vi "_LoPower_opt_fx.vi"(8 "ｘ":dbl, 9 "_LO_P_OPT":T1={"範囲配列"=[{"Start"=1.0, "Stop"=4.0, "Step"=0.05, "ｂｙ"="NEL VG"}, {"Start"=0.0, "Stop"=100.0, "Step"=4.0, "ｂｙ"="Motor"}, {"Start"=0.0, "Stop"=2.5, "Step"=0.1, "ｂｙ"="WCA VD"}], "Optimize"=0, "file_name"="LP_914.0_Tmin_100519.csv", "Save?"=FALSE, "measure"=1, "current(uA)"=60.0, "wait(ms)"=0, "IFfrq(GHz)"=8.0, "aveg"=10, "SISparam option"=2} {"SISparam option" items=["Volt and Current", "Volt only"]; "measure" items=["Pmax (only HOT)", "Tmin (HOT/COLD)", "C current"]; "Optimize" items=["Sweep", "黄金分割"]; "範囲配列"."Step" format="%.2f"; "範囲配列"."Stop" format="%.2f"; "範囲配列"."Start" format="%.2f"}, 10 "Control":T2={"GPIB_ATT"="28", "6501Dev#"=1, "GPIB_SP"="18", "GPIB_PM"="13", "GPIB_DSA"="11", "GPIB_DMM (TPD)"="23", "GPIB_MPI"="2", "mortor設定"=[{"Axis"=0, "ID"=0, "HIspeed"=200.0, "LOspeed"=100.0, "ACCEL(ms)"=100.0, "Sratio"=50.0, "フリーラン\n"=TRUE, "文字列"="DSB HOT/COLD"}, {"Axis"=1, "ID"=0, "HIspeed"=4.0, "LOspeed"=4.0, "ACCEL(ms)"=100.0, "Sratio"=50.0, "フリーラン\n"=TRUE, "文字列"="SubMM Att"}], "DATAパス"=path "Z:/band10/Labview_ALMA/MIX95/test", "DBパス "=path "Z:/band10/Labview_ALMA/MIX95/test", "comment"="P1_Tmin", "ColdCarts"="003601", "Th"=295.0, "Tc"=77.0, "Set_SIS_volt"=2.1, "Offset"=0.0, "control"=0, "FreqLO"=800.0, "Set_Mag_Cur"=800.0, "MPI offset(mm)"=22.99, "HOT/COLD"=0} {"HOT/COLD" items=["DSB", "SBR", "GainComp"]; "control" items=["CLOSE LOOP", "OPEN LOOP", "Not Control"]}, 11 "Bias_LO_equip":T4={"Node address"=19, "CAN Interface"="CAN0", "Cartridge band"=10, "Slave Node in"={"Address"=19, "Serial Number"=[16, 71, 55, 76, 1, 8, 0, -15]}, "ObjHandle out"=196083776, "POL"=1, "sb"=1, "GPIB_SM (SIS S,V)"="24", "GPIB_DMM (SIS I)"="22", "GPIB_SM (MAG I) "="25", "GPIB_SG(LO)"="19", "GPIB_PW (PAMP) "="6", "GPIB_TMP1(8ch)"="12", "GPIB_TMP2(2ch)  "="13", "WCA_avg"=10, "Rsen"=10.0, "BiasModule"=1, "LOModule "=2, "WCA_LO_FREQ_SET"={"YTO Low freq. [GHz]"=14.42, "YTO High freq. [GHz]"=17.7, "Kvco"=1, "Lock Pol."=0, "SET LO FREQ"=100.0, "Multiplier"=6.0, "YTO (HEX)"=2805, "YTO coarse( FREQ)"=16.666666, "NULL PLL INTEGRATOR"=TRUE}, "Res for"=0} {"Res for" items=["none", "series res", "parallel res"]; "WCA_LO_FREQ_SET"."YTO coarse( FREQ)" min=25 max=150 step=0.0001 format="%.3f"; "WCA_LO_FREQ_SET"."Multiplier" min=3 max=6 step=3; "WCA_LO_FREQ_SET"."SET LO FREQ" min=25 max=150 step=0.0001 format="%.3f"; "WCA_LO_FREQ_SET"."Lock Pol." items=["Lower", "Upper"]; "WCA_LO_FREQ_SET"."Kvco" items=["7.5MHz/V", "15MHz/V"]; "WCA_LO_FREQ_SET"."YTO High freq. [GHz]" format="%.3f"; "WCA_LO_FREQ_SET"."YTO Low freq. [GHz]" format="%.3f"; "LOModule" items=["Manual", "B10Lab LO", "WCA LO"]; "BiasModule" items=["B10Lab Bias", "WCA BiasModule"]; "Slave Node in"."Serial Number" format="%.0x"; "Slave Node in"."Address" format="%.0x"; "Cartridge band" max=10 step=1; "Node address" format="%.0x"}) -> (0 "出力配列":dbl[](array[numeric]), 3 "fx":dbl)   [LabVIEW 2017]
uses:
  <vilib>/express/express arith-compare/Formula/XNode/ExpressFormulaBlockNode.xnode
panel:
  in  "motor":T3={"Axis"=0, "ID"=0, "HIspeed"=100.0, "LOspeed"=100.0, "ACCEL(ms)"=100.0, "Sratio"=50.0, "移動距離"=50.0, "フリーラン\n"=FALSE}
  out "電圧":dbl
  out "Trx":dbl
  out "Ph":dbl
  out "Pc":dbl
  out "電流":dbl
  # "LO freq. [GHz]"
  # "YTO LOW\n/High Freq."
  # "ZERO Intgrtr"
  # "Node Address"
  # "Serial Number"
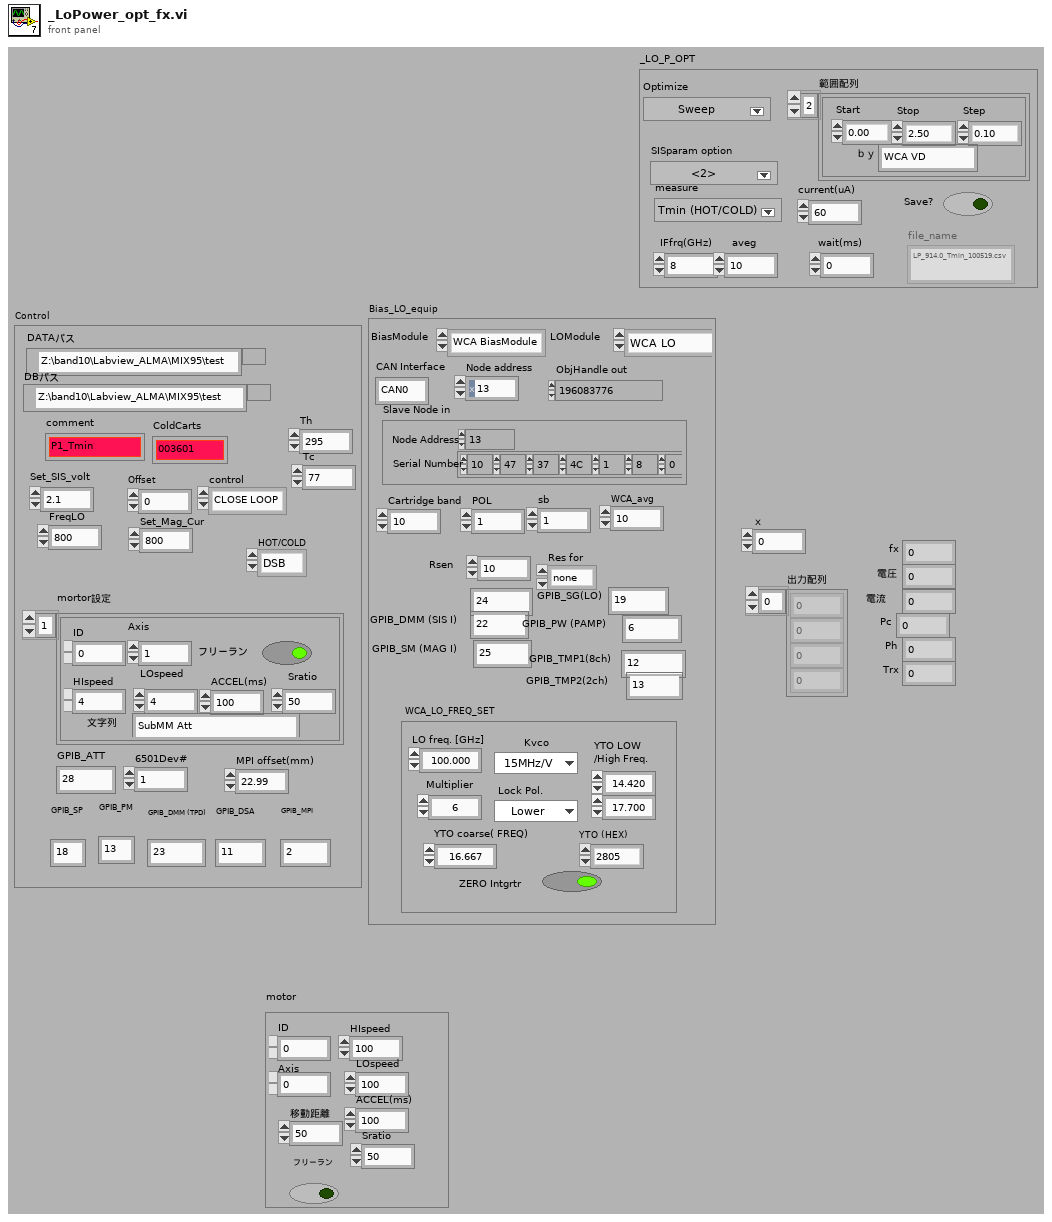
[diagram p1: front panel]
types:
  T1 = cluster{"範囲配列":cluster{"Start":dbl, "Stop":dbl, "Step":dbl, "ｂｙ":string}[], "Optimize":u16, "file_name":string, "Save?":bool, "measure":u16, "current(uA)":dbl, "wait(ms)":i32, "IFfrq(GHz)":dbl, "aveg":i32, "SISparam option":u16}
  T2 = cluster{"GPIB_ATT":string, "6501Dev#":i16, "GPIB_SP":string, "GPIB_PM":string, "GPIB_DSA":string, "GPIB_DMM (TPD)":string, "GPIB_MPI":string, "mortor設定":cluster{"Axis":i16, "ID":i16, "HIspeed":dbl, "LOspeed":dbl, "ACCEL(ms)":dbl, "Sratio":dbl, "フリーラン\n":bool, "文字列":string}[], "DATAパス":path, "DBパス ":path, "comment":string, "ColdCarts":string, "Th":dbl, "Tc":dbl, "Set_SIS_volt":dbl, "Offset":dbl, "control":u16, "FreqLO":dbl, "Set_Mag_Cur":dbl, "MPI offset(mm)":dbl, "HOT/COLD":u16}
  T3 = cluster{"Axis":i16, "ID":i16, "HIspeed":dbl, "LOspeed":dbl, "ACCEL(ms)":dbl, "Sratio":dbl, "移動距離":dbl, "フリーラン\n":bool}
  T4 = cluster{"Node address":u16, "CAN Interface":string, "Cartridge band":u32, "Slave Node in":cluster{"Address":i16, "Serial Number":i8[]}, "ObjHandle out":u32, "POL":u32, "sb":u32, "GPIB_SM (SIS S,V)":string, "GPIB_DMM (SIS I)":string, "GPIB_SM (MAG I) ":string, "GPIB_SG(LO)":string, "GPIB_PW (PAMP) ":string, "GPIB_TMP1(8ch)":string, "GPIB_TMP2(2ch)  ":string, "WCA_avg":i32, "Rsen":dbl, "BiasModule":u16, "LOModule ":u16, "WCA_LO_FREQ_SET":cluster{"YTO Low freq. [GHz]":sgl, "YTO High freq. [GHz]":sgl, "Kvco":u16, "Lock Pol.":u16, "SET LO FREQ":sgl, "Multiplier":sgl, "YTO (HEX)":u16, "YTO coarse( FREQ)":sgl, "NULL PLL INTEGRATOR":bool}, "Res for":u16}
  T5 = cluster{"Axis":i16, "ID":i16, "HIspeed":dbl, "LOspeed":dbl, "ACCEL(ms)":dbl, "Sratio":dbl, "フリーラン\n":bool, "文字列":string}[]
  T6 = cluster{"Axis":i16, "ID":i16, "HIspeed":dbl, "LOspeed":dbl, "ACCEL(ms)":dbl, "Sratio":dbl, "フリーラン\n":bool, "文字列":string}
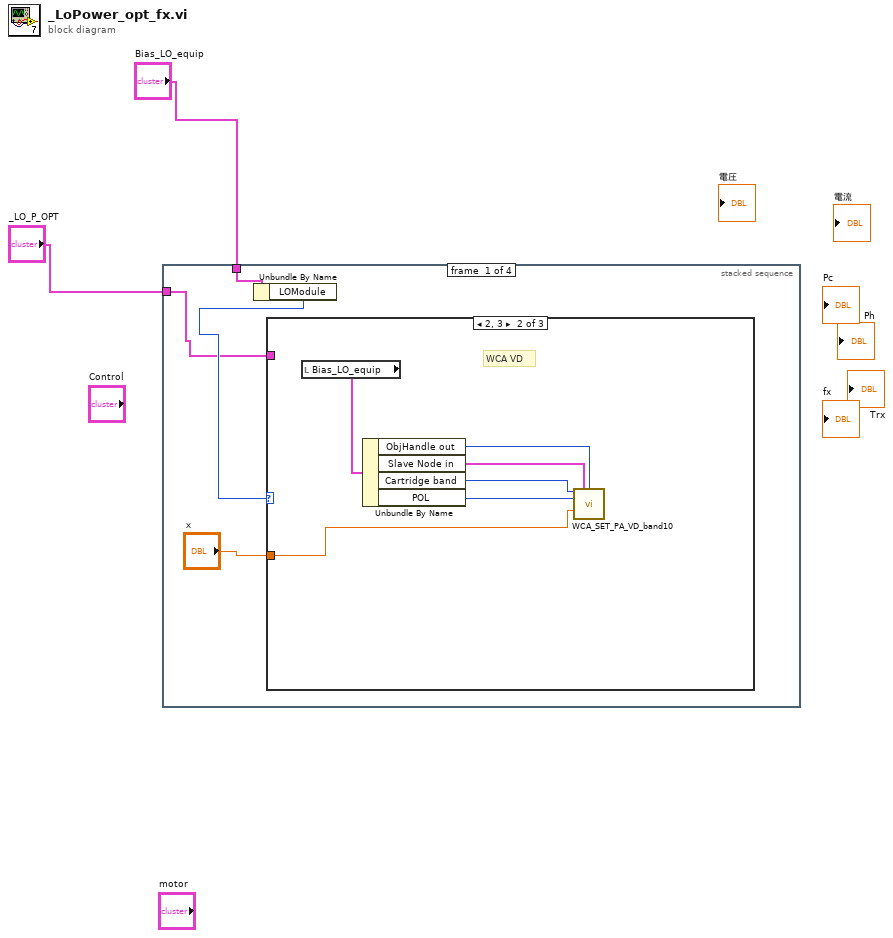
[diagram p0: block diagram]
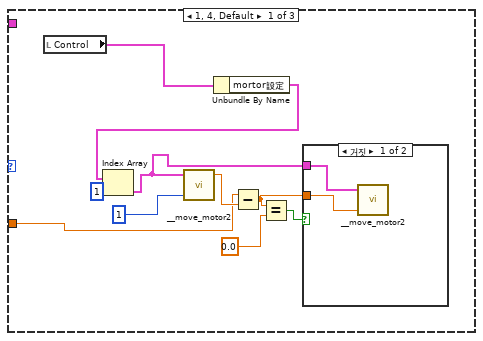
[diagram p2: hidden frame]
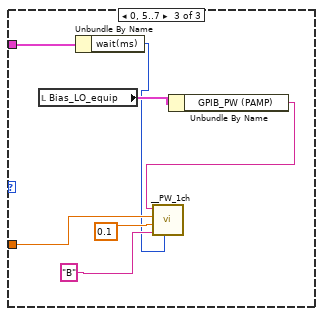
[diagram p4: hidden frame]
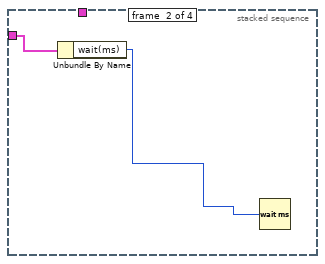
[diagram p5: hidden frame]
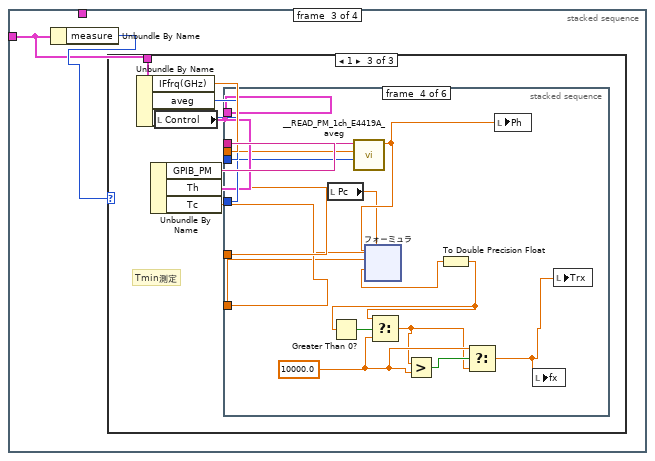
[diagram p6: hidden frame]
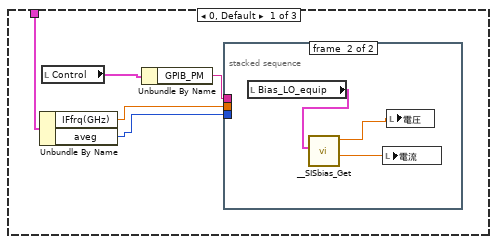
[diagram p7: hidden frame]
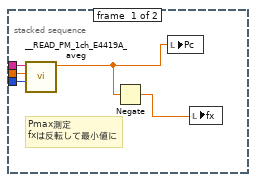
[diagram p8: hidden frame]
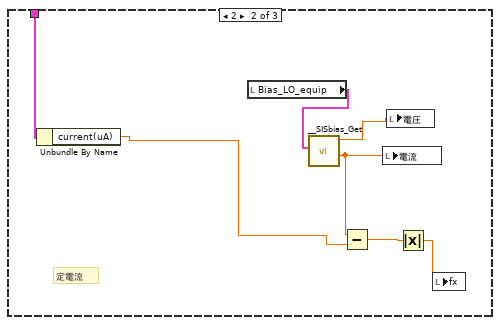
[diagram p9: hidden frame]
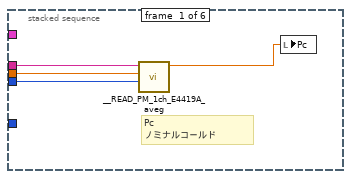
[diagram p10: hidden frame]
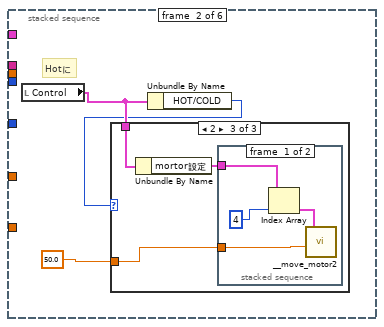
[diagram p11: hidden frame]
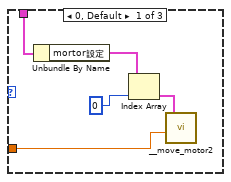
[diagram p12: hidden frame]
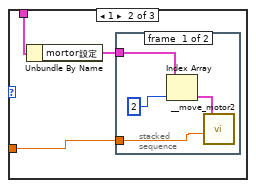
[diagram p13: hidden frame]
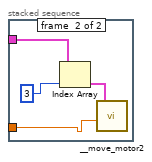
[diagram p14: hidden frame]
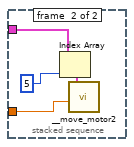
[diagram p15: hidden frame]
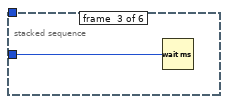
[diagram p16: hidden frame]
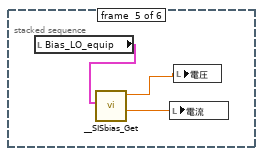
[diagram p17: hidden frame]
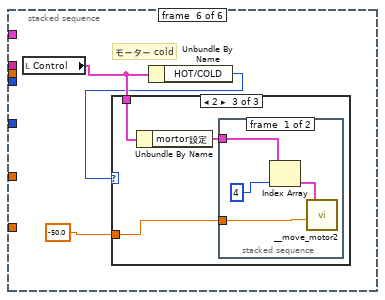
[diagram p18: hidden frame]
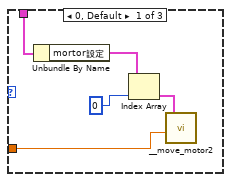
[diagram p19: hidden frame]
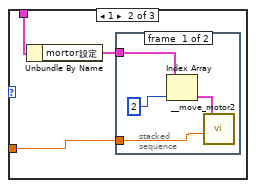
[diagram p20: hidden frame]
diagram:
  n1 = stacked-sequence {
    tunnel: "_LO_P_OPT" -> [w4 w33 w34 _]
    tunnel: "Bias_LO_equip" -> [w3 _ _ _]
    frame #0 {
      n2 = Unbundle By Name(w3) -> ("LOModule"=w5:u16)
      n3 = case shown="2, 3" w5 {
        tunnel: "ｘ" -> [w11 w19 w29]
        tunnel: w4 -> [_ _ w26]
        frame 1, 4, Default {
          n4 = local read "Control"() -> (w14:T2)
          n5 = Unbundle By Name(w14) -> ("mortor設定"=w16:T5)
          n6 = Index Array(array=w16, index=1) -> (element=w8:T6)
          n7 = call "__move_motor2.vi"("Moving distance"=1, "motor setup"=w8) -> ("counter"=w12:dbl)  [unwired: 2 in, 1 out]
          n8 = Subtract(x=w11, y=w12) -> (x-y=w7:dbl)
          n9 = Equal?(x=w7, y=0.0) -> (x = y?=w9:bool)
          n10 = case shown="거짓" w9 {
            tunnel: w8 -> [w18 _]
            tunnel: w7 -> [w17 _]
            frame False {
              n11 = call "__move_motor2.vi"("Moving distance"=w17, "motor setup"=w18) -> ()  [unwired: 2 in, 2 out]
            }
            frame True {
            }
          }
        }
        frame 2, 3 {
          # "WCA VD"
          n12 = local read "Bias_LO_equip"() -> (w24:T4)
          n13 = Unbundle By Name(w24) -> ("ObjHandle out"=w22:u32, "Slave Node in"=w23:cluster{"Address":i16, "Serial Number":i8[]}, "Cartridge band"=w21:u32, "POL"=w20:u32)
          n14 = call "WCA_SET_PA_VD_band10.vi"("Cartridge Band"=w21, "Slave Node in"=w23, "ObjHandle in"=w22, "POL（P0、P1）"=w20, "SET_PA_VD"=w19) -> ()  [unwired: 9 in, 2 out]
        }
        frame 0, 5..7 {
          n15 = local read "Bias_LO_equip"() -> (w31:T4)
          n16 = Unbundle By Name(w26) -> ("wait(ms)"=w25:i32)
          n17 = Unbundle By Name(w31) -> ("GPIB_PW (PAMP)"=w30:string)
          n18 = call "__PW_1ch.vi"("Wait(ms)"=w25, "Ch（A,B,C,D）"="B", "A(A)"=0.1, "V(V)"=w29, "GPIB"=w30) -> ()  [unwired: 5 in, 2 out]
        }
      }
    }
    frame #1 {
      n19 = Unbundle By Name(w33) -> ("wait(ms)"=w32:i32)
      n20 = Wait (ms)(milliseconds to wait=w32) -> ()  [unwired: 1 out]
    }
    frame #2 {
      n21 = Unbundle By Name(w34) -> ("measure"=w35:u16)
      n22 = case shown="1" w35 {
        tunnel: w34 -> [w38 w55 w62]
        frame 0, Default {
          n23 = Unbundle By Name(w38) -> ("IFfrq(GHz)"=w37:dbl, "aveg"=w36:i32)
          n24 = local read "Control"() -> (w40:T2)
          n25 = Unbundle By Name(w40) -> ("GPIB_PM"=w39:string)
          n26 = stacked-sequence {
            tunnel: w39 -> [w45 _]
            tunnel: w37 -> [w44 _]
            tunnel: w36 -> [w43 _]
            frame #0 {
              # "Pmax測定\nfxは反転して最小値に"
              n27 = call "__READ_PM_1ch_E4419A_aveg.VI"("aveg"=w43, "frq(GHz)"=w44, "GPIB"=w45) -> ("chA"=w42:dbl)  [unwired: 4 in]
              n28 = Negate(x=w42) -> (-x=w41:dbl)
              n29 = local write "Pc"(w42) -> ()
              n30 = local write "fx"(w41) -> ()
            }
            frame #1 {
              n31 = local read "Bias_LO_equip"() -> (w48:T4)
              n32 = call "__SISbias_Get.vi"("Bias_LO_equip"=w48) -> ("Get_I(uA)"=w47:dbl, "Get_V(mV)"=w46:dbl)  [unwired: 8 in, 1 out]
              n33 = local write "電流"(w47) -> ()
              n34 = local write "電圧"(w46) -> ()
            }
          }
        }
        frame 2 {
          # "定電流"
          n35 = Unbundle By Name(w55) -> ("current(uA)"=w51:dbl)
          n36 = local read "Bias_LO_equip"() -> (w54:T4)
          n37 = call "__SISbias_Get.vi"("Bias_LO_equip"=w54) -> ("Get_I(uA)"=w52:dbl, "Get_V(mV)"=w53:dbl)  [unwired: 8 in, 1 out]
          n38 = Subtract(x=w52, y=w51) -> (x-y=w50:dbl)
          n39 = local write "電流"(w52) -> ()
          n40 = local write "電圧"(w53) -> ()
          n41 = Absolute Value(x=w50) -> (abs(x)=w49:dbl)
          n42 = local write "fx"(w49) -> ()
        }
        frame 1 {
          # "Tmin測定"
          n43 = Unbundle By Name(w62) -> ("IFfrq(GHz)"=w61:dbl, "aveg"=w60:i32, "wait(ms)"=w59:i32)
          n44 = local read "Control"() -> (w58:T2)
          n45 = Unbundle By Name(w58) -> ("GPIB_PM"=w63:string, "Th"=w57:dbl, "Tc"=w56:dbl)
          n46 = stacked-sequence {
            tunnel: w63 -> [w67 _ _ w112 _ _]
            tunnel: w61 -> [w66 _ _ w111 _ _]
            tunnel: w60 -> [w65 _ _ w110 _ _]
            tunnel: w59 -> [_ _ w98 _ _ _]
            tunnel: w57 -> [_ _ _ w109 _ _]
            tunnel: w56 -> [_ _ _ w108 _ _]
            tunnel: w58 -> [_ _ _ _ _ _]
            frame #0 {
              # "Pc\nノミナルコールド"
              n47 = call "__READ_PM_1ch_E4419A_aveg.VI"("aveg"=w65, "frq(GHz)"=w66, "GPIB"=w67) -> ("chA"=w64:dbl)  [unwired: 4 in]
              n48 = local write "Pc"(w64) -> ()
            }
            frame #1 {
              # "Hotに"
              n49 = local read "Control"() -> (w70:T2)
              n50 = Unbundle By Name(w70) -> ("HOT/COLD"=w69:u16)
              n51 = case shown="2" w69 {
                tunnel: w70 -> [w74 w78 w89]
                tunnel: 50.0 -> [w71 w76 w87]
                frame 0, Default {
                  n52 = Unbundle By Name(w74) -> ("mortor設定"=w73:T5)
                  n53 = Index Array(array=w73, index=0) -> (element=w72:T6)
                  n54 = call "__move_motor2.vi"("Moving distance"=w71, "motor setup"=w72) -> ()  [unwired: 2 in, 2 out]
                }
                frame 1 {
                  n55 = Unbundle By Name(w78) -> ("mortor設定"=w77:T5)
                  n56 = stacked-sequence {
                    tunnel: w77 -> [w81 w85]
                    tunnel: w76 -> [w79 w83]
                    frame #0 {
                      n57 = Index Array(array=w81, index=2) -> (element=w80:T6)
                      n58 = call "__move_motor2.vi"("Moving distance"=w79, "motor setup"=w80) -> ()  [unwired: 2 in, 2 out]
                    }
                    frame #1 {
                      n59 = Index Array(array=w85, index=3) -> (element=w84:T6)
                      n60 = call "__move_motor2.vi"("Moving distance"=w83, "motor setup"=w84) -> ()  [unwired: 2 in, 2 out]
                    }
                  }
                }
                frame 2 {
                  n61 = Unbundle By Name(w89) -> ("mortor設定"=w88:T5)
                  n62 = stacked-sequence {
                    tunnel: w88 -> [w92 w96]
                    tunnel: w87 -> [w90 w94]
                    frame #0 {
                      n63 = Index Array(array=w92, index=4) -> (element=w91:T6)
                      n64 = call "__move_motor2.vi"("Moving distance"=w90, "motor setup"=w91) -> ()  [unwired: 2 in, 2 out]
                    }
                    frame #1 {
                      n65 = Index Array(array=w96, index=5) -> (element=w95:T6)
                      n66 = call "__move_motor2.vi"("Moving distance"=w94, "motor setup"=w95) -> ()  [unwired: 2 in, 2 out]
                    }
                  }
                }
              }
            }
            frame #2 {
              n67 = Wait (ms)(milliseconds to wait=w98) -> ()  [unwired: 1 out]
            }
            frame #3 {
              w101 = 10000.0
              # "Pｈ"
              n68 = local read "Pc"() -> (w105:dbl)
              n69 = call "__READ_PM_1ch_E4419A_aveg.VI"("aveg"=w110, "frq(GHz)"=w111, "GPIB"=w112) -> ("chA"=w106:dbl)  [unwired: 4 in]
              n70 = xnode "フォーミュラ"("ph"=w106, "pc"=w105, "th"=w109, "tc"=w108) -> ("結果"=w107:dbl)  [unwired: 1 in, 1 out]
              n71 = To Double Precision Float(number=w107) -> (double precision float=w104:dbl)
              n72 = Greater Than 0?(x=w104) -> (x > 0?=w103:bool)
              n73 = Select(t=w104, s=w103, f=w101) -> (s? t:f=w100:dbl)
              n74 = Greater?(x=w100, y=w101) -> (0:w102:bool)
              n75 = Select(t=w101, s=w102, f=w100) -> (s? t:f=w99:dbl)
              n76 = local write "Ph"(w106) -> ()
              n77 = local write "fx"(w99) -> ()
              n78 = local write "Trx"(w99) -> ()
            }
            frame #4 {
              n79 = local read "Bias_LO_equip"() -> (w129:T4)
              n80 = call "__SISbias_Get.vi"("Bias_LO_equip"=w129) -> ("Get_I(uA)"=w128:dbl, "Get_V(mV)"=w127:dbl)  [unwired: 8 in, 1 out]
              n81 = local write "電流"(w128) -> ()
              n82 = local write "電圧"(w127) -> ()
            }
            frame #5 {
              # "モーター cold"
              n83 = local read "Control"() -> (w132:T2)
              n84 = Unbundle By Name(w132) -> ("HOT/COLD"=w131:u16)
              n85 = case shown="2" w131 {
                tunnel: w132 -> [w136 w140 w151]
                tunnel: -50.0 -> [w133 w138 w149]
                frame 0, Default {
                  n86 = Unbundle By Name(w136) -> ("mortor設定"=w135:T5)
                  n87 = Index Array(array=w135, index=0) -> (element=w134:T6)
                  n88 = call "__move_motor2.vi"("Moving distance"=w133, "motor setup"=w134) -> ()  [unwired: 2 in, 2 out]
                }
                frame 1 {
                  n89 = Unbundle By Name(w140) -> ("mortor設定"=w139:T5)
                  n90 = stacked-sequence {
                    tunnel: w139 -> [w143 w147]
                    tunnel: w138 -> [w141 w145]
                    frame #0 {
                      n91 = Index Array(array=w143, index=2) -> (element=w142:T6)
                      n92 = call "__move_motor2.vi"("Moving distance"=w141, "motor setup"=w142) -> ()  [unwired: 2 in, 2 out]
                    }
                    frame #1 {
                      n93 = Index Array(array=w147, index=3) -> (element=w146:T6)
                      n94 = call "__move_motor2.vi"("Moving distance"=w145, "motor setup"=w146) -> ()  [unwired: 2 in, 2 out]
                    }
                  }
                }
                frame 2 {
                  n95 = Unbundle By Name(w151) -> ("mortor設定"=w150:T5)
                  n96 = stacked-sequence {
                    tunnel: w150 -> [w154 w158]
                    tunnel: w149 -> [w152 w156]
                    frame #0 {
                      n97 = Index Array(array=w154, index=4) -> (element=w153:T6)
                      n98 = call "__move_motor2.vi"("Moving distance"=w152, "motor setup"=w153) -> ()  [unwired: 2 in, 2 out]
                    }
                    frame #1 {
                      n99 = Index Array(array=w158, index=5) -> (element=w157:T6)
                      n100 = call "__move_motor2.vi"("Moving distance"=w156, "motor setup"=w157) -> ()  [unwired: 2 in, 2 out]
                    }
                  }
                }
              }
            }
          }
        }
      }
    }
    frame #3 {
      n101 = local read "Pc"() -> (w164:dbl)
      n102 = local read "Ph"() -> (w165:dbl)
      n103 = local read "電流"() -> (w166:dbl)
      n104 = local read "電圧"() -> (w167:dbl)
      n105 = local read "Trx"() -> (w163:dbl)
      n106 = local read "fx"() -> (w162:dbl)
      n107 = local read "ｘ"() -> (w160:dbl)
      n108 = Build Array(w160, w167, w166, w165, w164, w163, w162) -> (→"出力配列":dbl[])
    }
  }
